vi "Run.vi"(8 "error in (no error)":errorcluster, 11 "LUnit Test Case In":refnum<class "LUnit Test Case.lvclass">) -> (0 "error out":errorcluster, 1 "Done?":bool, 2 "Results":T1[](array[typedef]), 3 "LUnit Test Case Out":refnum<class "LUnit Test Case.lvclass">)   [LabVIEW 2020, in "LUnit Test Case.lvclass"]
doc: "Execute test and return result."
uses:
  LUnit Test Case.lvclass
  Result/Result.ctl
  Result/Status.ctl
  Result/Type.ctl
  LUnit Test Case.lvclass/LUnit Test Case.ctl
  Result/Result.lvlib
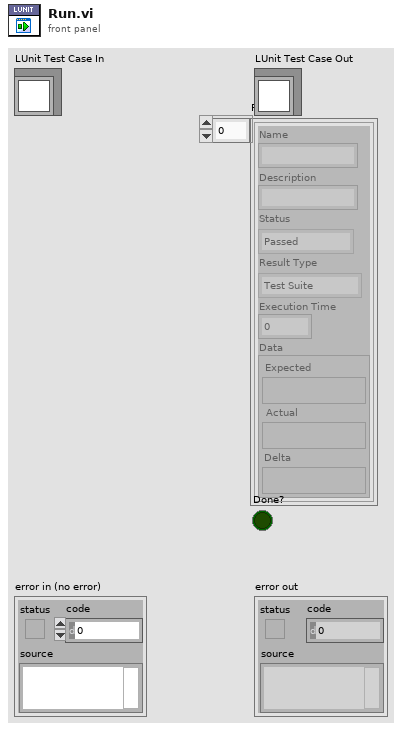
[diagram p1: front panel]
types:
  T1 = typedef "Result.lvlib/Result.ctl" = cluster{"Name":string, "Description":string, "Status":T2, "Result Type":T3, "Execution Time":dbl, "Data":cluster{"Expected":variant, "Actual":variant, "Delta":variant}}
  T2 = typedef "Result.lvlib/Status.ctl" = enum16{"", "Passed", "Failed", "Error", "Skipped", "Setup Error", "Broken", "Teardown Error"}
  T3 = typedef "Result.lvlib/Type.ctl" = enum16{"Test Case", "Test Suite", "Test Run", "Pass", "Fail", "Skip", "Pass if", "Fail if", "Pass if Error", "Fail if Error", "Pass if Equal", "Fail if Equal"}
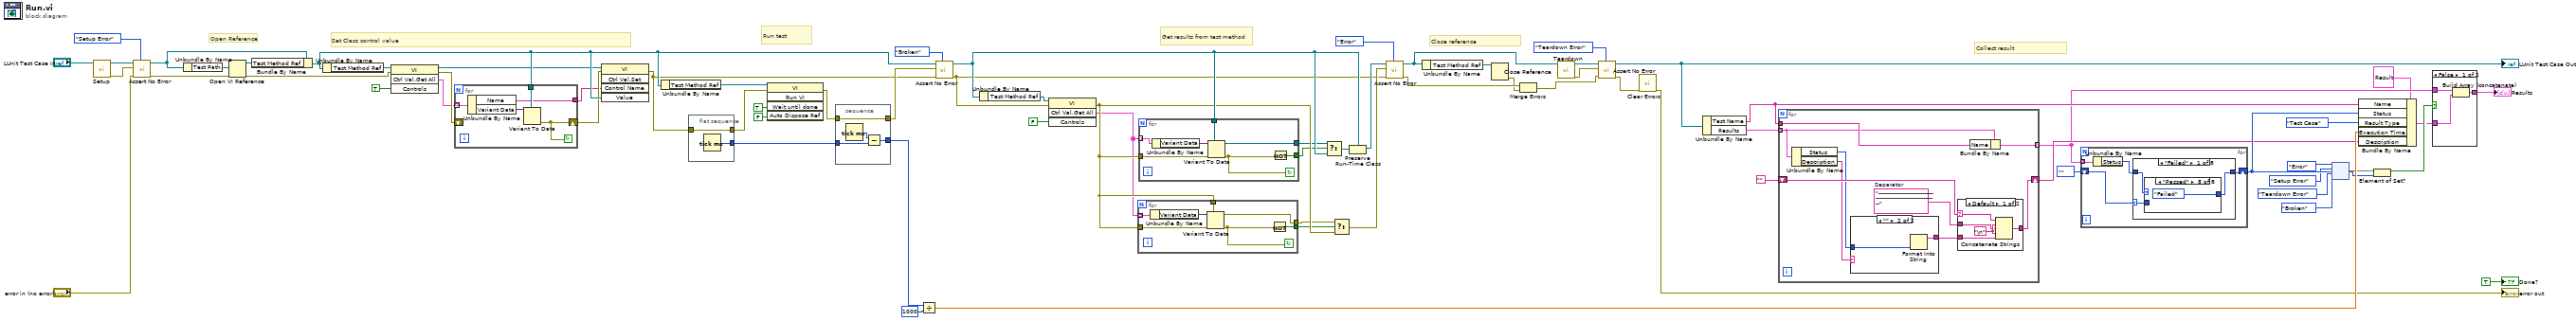
[diagram p0: block diagram]
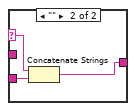
[diagram p2: hidden frame]
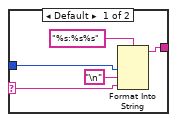
[diagram p3: hidden frame]
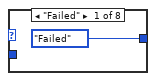
[diagram p4: hidden frame]
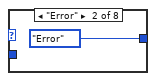
[diagram p5: hidden frame]
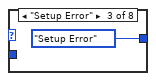
[diagram p6: hidden frame]
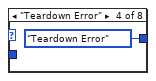
[diagram p7: hidden frame]
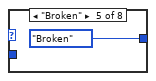
[diagram p8: hidden frame]
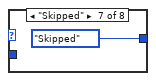
[diagram p10: hidden frame]
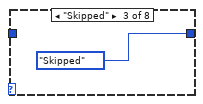
[diagram p12: hidden frame]
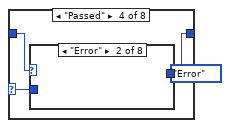
[diagram p13: hidden frame]
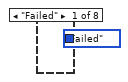
[diagram p14: hidden frame]
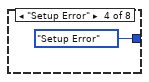
[diagram p16: hidden frame]
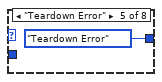
[diagram p17: hidden frame]
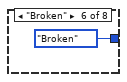
[diagram p18: hidden frame]
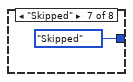
[diagram p19: hidden frame]
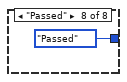
[diagram p20: hidden frame]
diagram:
  # "Collect result"
  # "Close reference"
  # "Get results from test method"
  # "Run test"
  # "Set Class control value"
  # "Open Reference"
  n1 = call-dynamic "Setup.vi"("LUnit Test Case In"="LUnit Test Case In") -> ("error out"=w64:errorcluster, "LUnit Test Case Out"=w69:refnum<class "LUnit Test Case.lvclass">)  [unwired: 9 in]
  n2 = call "Assert No Error.vi"("Status"=Status."Setup Error", "error In"="error in (no error)", "Assert error"=w64, "LUnit Test Case In"=w69) -> ("error out"=w70:errorcluster, "LUnit Test Case Out"=w68:refnum<class "LUnit Test Case.lvclass">)  [unwired: 6 in]
  n3 = Unbundle By Name(w68) -> ("Test Path"=w43:path)
  n4 = Open VI Reference(vi path=w43, error in (no error)=w70) -> (vi reference=w44:refnum<vi>, error out=w63:errorcluster)  [unwired: 4 in]
  n5 = Bundle By Name(cluster=w68, "Test Method Ref"=w44) -> (w62:refnum<class "LUnit Test Case.lvclass">)
  n6 = Unbundle By Name(w62) -> ("Test Method Ref"=w30:refnum<vi>)
  n7 = invoke on="Invoke Node" class="VI" method="Ctrl Val.Get All"(reference=w30, error in=w63, "Controls"=TRUE) -> (reference out=w29:refnum<vi>, error out=w31:errorcluster, "Get All Control Values Variant"=w27:cluster{"Name":string, "Variant Data":variant}[])  [unwired: 1 in, 1 out]
  n8 = for {
    tunnel: w27 -> [w78] mode=indexing
    tunnel: w62 -> [w76]
    tunnel: [w75] -> w26
    shift-right: [w74] -> w32
    shift-left: w31 -> [_]
    stop <- w74 continue-if-true
    n9 = Unbundle By Name(w78) -> ("Name"=w75:string, "Variant Data"=w77:variant)
    n10 = Variant To Data(type=w76, Variant=w77) -> (error out=w74:errorcluster)  [unwired: 1 in, 1 out]
  }
  n11 = invoke on="Invoke Node" class="VI" method="Ctrl Val.Set"(reference=w29, error in=w32, "Control Name"=w26, "Value"=w62) -> (error out=w57:errorcluster)  [unwired: 1 in, 4 out]
  n12 = Unbundle By Name(w62) -> ("Test Method Ref"=w36:refnum<vi>)
  n13 = flat-sequence {
    tunnel: w57 -> [w80]
    tunnel: [w80] -> w37
    tunnel: [w79] -> w39
    frame #0 {
      n14 = Tick Count (ms)() -> (millisecond timer value=w79:u32)
    }
  }
  n15 = invoke class="VI" method="Run VI"(reference=w36, error in=w37, "Wait until done"=TRUE ("Wait Until Done"), "Auto Dispose Ref"=FALSE ("Auto Dispose Reference")) -> (error out=w38:errorcluster)  [unwired: 1 in, 4 out]
  n16 = stacked-sequence {
    tunnel: [w82] -> w58
    tunnel: [w83] -> w40
    tunnel: w38 -> [w82]
    tunnel: w39 -> [w81]
    frame #0 {
      n17 = Tick Count (ms)() -> (millisecond timer value=w84:u32)
      n18 = Subtract(x=w84, y=w81) -> (x-y=w83:u32)
    }
  }
  n19 = Divide(x=w40, y=u32 1000) -> (x/y=w72:dbl)
  n20 = call "Assert No Error.vi"("Status"=Status."Broken", "error In"=w57, "Assert error"=w58, "LUnit Test Case In"=w62) -> ("error out"=w52:errorcluster, "LUnit Test Case Out"=w60:refnum<class "LUnit Test Case.lvclass">)  [unwired: 6 in]
  n21 = Unbundle By Name(w60) -> ("Test Method Ref"=w21:refnum<vi>)
  n22 = invoke on="Invoke Node" class="VI" method="Ctrl Val.Get All"(reference=w21, error in=w52, "Controls"=FALSE) -> (error out=w25:errorcluster, "Get All Control Values Variant"=w22:cluster{"Name":string, "Variant Data":variant}[])  [unwired: 1 in, 2 out]
  n23 = for {
    tunnel: w22 -> [w91] mode=indexing
    tunnel: w25 -> [w89]
    tunnel: [w85] -> w23
    tunnel: [w87] -> w24
    tunnel: w25 -> [w86]
    stop <- w88 continue-if-true
    n24 = Unbundle By Name(w91) -> ("Variant Data"=w90:variant)
    n25 = Variant To Data(error in=w86, type=w89, Variant=w90) -> (data=w87:errorcluster, error out=w88:errorcluster)
    n26 = Not(x=w88) -> (.not. x?=w85:bool)
  }
  n27 = for {
    tunnel: w22 -> [w98] mode=indexing
    tunnel: w60 -> [w96]
    tunnel: [w92] -> w19
    tunnel: [w94] -> w20
    tunnel: w25 -> [w93]
    stop <- w95 continue-if-true
    n28 = Unbundle By Name(w98) -> ("Variant Data"=w97:variant)
    n29 = Variant To Data(error in=w93, type=w96, Variant=w97) -> (data=w94:refnum<class "LUnit Test Case.lvclass">, error out=w95:errorcluster)
    n30 = Not(x=w95) -> (.not. x?=w92:bool)
  }
  n31 = Select(t=w20, s=w19, f=w60) -> (s? t:f=w17:refnum<class "LUnit Test Case.lvclass">)
  n32 = Select(t=w24, s=w23, f=w25) -> (s? t:f=w53:errorcluster)
  n33 = Preserve Run-Time Class(object in=w17, 2:w60) -> (object out=w56:refnum<class "LUnit Test Case.lvclass">)  [unwired: 1 in, 1 out]
  n34 = call "Assert No Error.vi"("Status"=Status."Error", "error In"=w52, "Assert error"=w53, "LUnit Test Case In"=w56) -> ("error out"=w55:errorcluster, "LUnit Test Case Out"=w61:refnum<class "LUnit Test Case.lvclass">)  [unwired: 6 in]
  n35 = Unbundle By Name(w61) -> ("Test Method Ref"=w42:refnum<vi>)
  n36 = Close Reference(reference=w42) -> (error out=w41:errorcluster)  [unwired: 1 in]
  n37 = Merge Errors(w55, w41) -> (w48:errorcluster)
  n38 = call-dynamic "Teardown.vi"("LUnit Test Case In"=w61) -> ("error out"=w49:errorcluster, "LUnit Test Case Out"=w51:refnum<class "LUnit Test Case.lvclass">)  [unwired: 9 in]
  n39 = call "Assert No Error.vi"("Status"=Status."Teardown Error", "error In"=w48, "Assert error"=w49, "LUnit Test Case In"=w51) -> ("error out"=w66:errorcluster, "LUnit Test Case Out"=w45:refnum<class "LUnit Test Case.lvclass">)  [unwired: 6 in]
  "LUnit Test Case Out" <- w45
  n40 = call <vilib>:"Clear Errors.vi"("error in (no error)"=w66) -> ("error out"=→"error out":errorcluster)  [unwired: 5 in, 1 out]
  n41 = Unbundle By Name(w45) -> ("Test Name"=w14:string, "Results"=w1:T1[])
  n42 = for {
    tunnel: w1 -> [w104] mode=indexing
    tunnel: w14 -> [w107]
    tunnel: [w106] -> w3 mode=indexing
    shift-right: [w101] -> w7
    shift-left: "" ("Input String") -> [w105]
    w99 = "-------------------------------------------------------------"  # Separator
    n43 = Unbundle By Name(w104) -> ("Status"=w103:T2, "Description"=w102:string)
    n44 = case shown="\"\"" w102 {
      selector: w102 -> [w119 _]
      tunnel: w103 -> [w120 w122]
      tunnel: [w118 w121] -> w100
      frame Default {
        n45 = Format Into String(format string="%s:%s%s", w120, "\n", w119) -> (resulting string=w118:string)  [unwired: 2 in, 1 out]
      }
      frame "" {
        n46 = Format Into String(w122) -> (resulting string=w121:string)  [unwired: 3 in, 1 out]
      }
    }
    n47 = case shown="Default" w105 {
      selector: w105 -> [w111 w113]
      tunnel: w100 -> [w109 w115]
      tunnel: w99 -> [w108 _]
      tunnel: [w112 w114] -> w101
      frame Default {
        w110 = "\n"
        n48 = Concatenate Strings(w111, w110, w108, w110, w109) -> (w112:string)
      }
      frame "" {
        n49 = Concatenate Strings(w113, w115) -> (w114:string)
      }
    }
    n50 = Bundle By Name(cluster=w104, "Name"=w107) -> (w106:T1)
  }
  n51 = for {
    tunnel: w3 -> [w126] mode=indexing
    shift-right: [w124] -> w16
    shift-left: Status."" ("Current") -> [w125]
    n52 = Unbundle By Name(w126) -> ("Status"=w123:T2)
    n53 = case shown="\"Failed\"" w125 {
      selector: w125 -> [w127 _ _ w140 w151 _ _ _]
      tunnel: w123 -> [w129 w138 _ w142 w152 w157 w161 w165]
      tunnel: [w128 w138 Status."Skipped" ("Merged Status") w141 w153 w158 w162 w166] -> w124
      frame "Failed" {
        n54 = case shown="\"Passed\"" w129 {
          tunnel: [Status."Failed" ("Merged Status") Status."Error" ("Merged Status") Status."Setup Error" ("Merged Status") Status."Teardown Error" ("Merged Status") Status."Broken" ("Merged Status") w135 Status."Skipped" ("Merged Status") Status."Failed" ("Merged Status")] -> w128
          tunnel: w127 -> [_ _ _ _ _ w135 _ _]
          frame "Failed" {
          }
          frame "Error" {
          }
          frame "Setup Error" {
          }
          frame "Teardown Error" {
          }
          frame "Broken" {
          }
          frame "" {
          }
          frame "Skipped" {
          }
          frame "Passed" {
          }
        }
      }
      frame "" {
      }
      frame "Skipped" {
      }
      frame "Passed" {
        n55 = case shown="\"Error\"" w142 {
          tunnel: [Status."Failed" ("Merged Status") Status."Error" ("Merged Status") w145 Status."Setup Error" ("Merged Status") Status."Teardown Error" ("Merged Status") Status."Broken" ("Merged Status") Status."Skipped" ("Merged Status") Status."Passed" ("Merged Status")] -> w141
          tunnel: w140 -> [_ _ w145 _ _ _ _ _]
          frame "Failed" {
          }
          frame "Error" {
          }
          frame "" {
          }
          frame "Setup Error" {
          }
          frame "Teardown Error" {
          }
          frame "Broken" {
          }
          frame "Skipped" {
          }
          frame "Passed" {
          }
        }
      }
      frame "Error" {
        n56 = case shown="Default" w152 {
          tunnel: [Status."Skipped" ("Merged Status") w155 Status."Error" ("Merged Status")] -> w153
          tunnel: w151 -> [_ w155 _]
          frame "Skipped" {
          }
          frame "" {
          }
          frame Default {
          }
        }
      }
      frame "Setup Error" {
        n57 = case shown="Default" w157 {
          tunnel: [Status."Skipped" ("Merged Status") Status."Setup Error" ("Merged Status")] -> w158
          frame "Skipped" {
          }
          frame Default {
          }
        }
      }
      frame "Broken" {
        n58 = case shown="Default" w161 {
          tunnel: [Status."Broken" ("Merged Status") Status."Setup Error" ("Merged Status")] -> w162
          frame Default {
          }
          frame "Setup Error" {
          }
        }
      }
      frame "Teardown Error" {
        n59 = case shown="\"Skipped\"" w165 {
          tunnel: [Status."Skipped" ("Merged Status") Status."Teardown Error" ("Merged Status")] -> w166
          frame "Skipped" {
          }
          frame Default {
          }
        }
      }
    }
  }
  n60 = node(Status."Error" ("Status"), Status."Setup Error" ("Status"), Status."Teardown Error" ("Status"), Status."Broken" ("Status")) -> (w12:set{T2})
  n61 = Bundle By Name(cluster=T1 {"Name"="", "Description"="", "Status"=enum."Passed", "Result Type"=enum."Test Case", "Execution Time"=0.0, "Data"={"Expected"=variant, "Actual"=variant, "Delta"=variant}} ("Results"), "Name"=w14, "Status"=w16, "Result Type"=Type."Test Case", "Execution Time"=w72, "Description"=w7) -> (w4:T1)
  n62 = Element of Set?(10:w16, 11:w12) -> (3:w13:bool)
  n63 = case shown="False" w13 {
    tunnel: w3 -> [w171 w172]
    tunnel: [w170 w172] -> w73
    tunnel: w4 -> [w169 _]
    frame False {
      n64 = Build Array (concatenate)(w171, w169) -> (w170:T1[])
    }
    frame True {
    }
  }
  "Results" <- w73
  "Done?" <- TRUE ("Done?")
